vi "Modbus Master Simple.vi"() -> ()   [LabVIEW 2017]
uses:
  <vilib>/NI/Modbus Library/API/Master/Set Read Timeout.vi
  <vilib>/NI/Modbus Library/API/Read Transmission Data Unit.vi
  <vilib>/NI/Modbus Library/API/Write Transmission Data Unit.vi
  <vilib>/NI/Modbus Library/Transmission Data Unit/Write read operation timeout.vi
  <vilib>/NI/Modbus Library/API/Wrapper/Create Serial Master.vi
  <vilib>/NI/Modbus Library/API/Master/Modbus Master.lvclass
  <vilib>/NI/Modbus Library/API/Wrapper/API Main.lvlib
panel:
  in  "Read Timeout":i32=500
  out "Array 5":errorcluster[](array[cluster])
  in  "Inputs":T1(array[cluster])=[{"Inputs"=[0, 0, 0, 0], "Address"=0, "Number"=4}] {"Inputs" scale=0.0..65535.0}
  in  "Stop Button":bool
  out "Array 4":errorcluster[](array[cluster])
  out "Array 3":errorcluster[](array[cluster])
  out "Array 2":errorcluster[](array[cluster])
  out "Array":errorcluster[](array[cluster])=[{"status"=FALSE, "code"=0, "source"=""}, {"status"=TRUE, "code"=538183, "source"="<APPEND>Function 15"}, {"status"=TRUE, "code"=538183, "source"="<APPEND>Function 15"}]
  out "error out":errorcluster
  in  "Write Holding Reg":T2(array[cluster])=[{"Registers"=[1, 2], "Address"=4, "Number"=2}]
  in  "Read Holding Reg":T2(array[cluster])=[{"Registers"=[0, 0], "Address"=0, "Number"=2}]
  in  "DIscrete Inputs":T3(array[cluster])=[{"Inputs"=[TRUE, FALSE, TRUE, FALSE], "Address"=0, "Number"=4}]
  in  "Coils":cluster{"Coils":bool[], "Address":u16}[](array[cluster])=[{"Coils"=[TRUE, TRUE, TRUE, TRUE, TRUE], "Address"=0}, {"Coils"=[], "Address"=8}, {"Coils"=[], "Address"=16}] {"Address" format="%x"}
  in  "Update Period(ms)":u64=200
  in  "baud rate":u32=9600
  in  "VISA resource name":refnum<visa-resource-name>="COM13"
  in  "unit ID":u8=1
  in  "serial type":enum16{"RTU", "ASCII"}(ring)=enum."ASCII"
  in  "Connect":bool
  # "Slave"
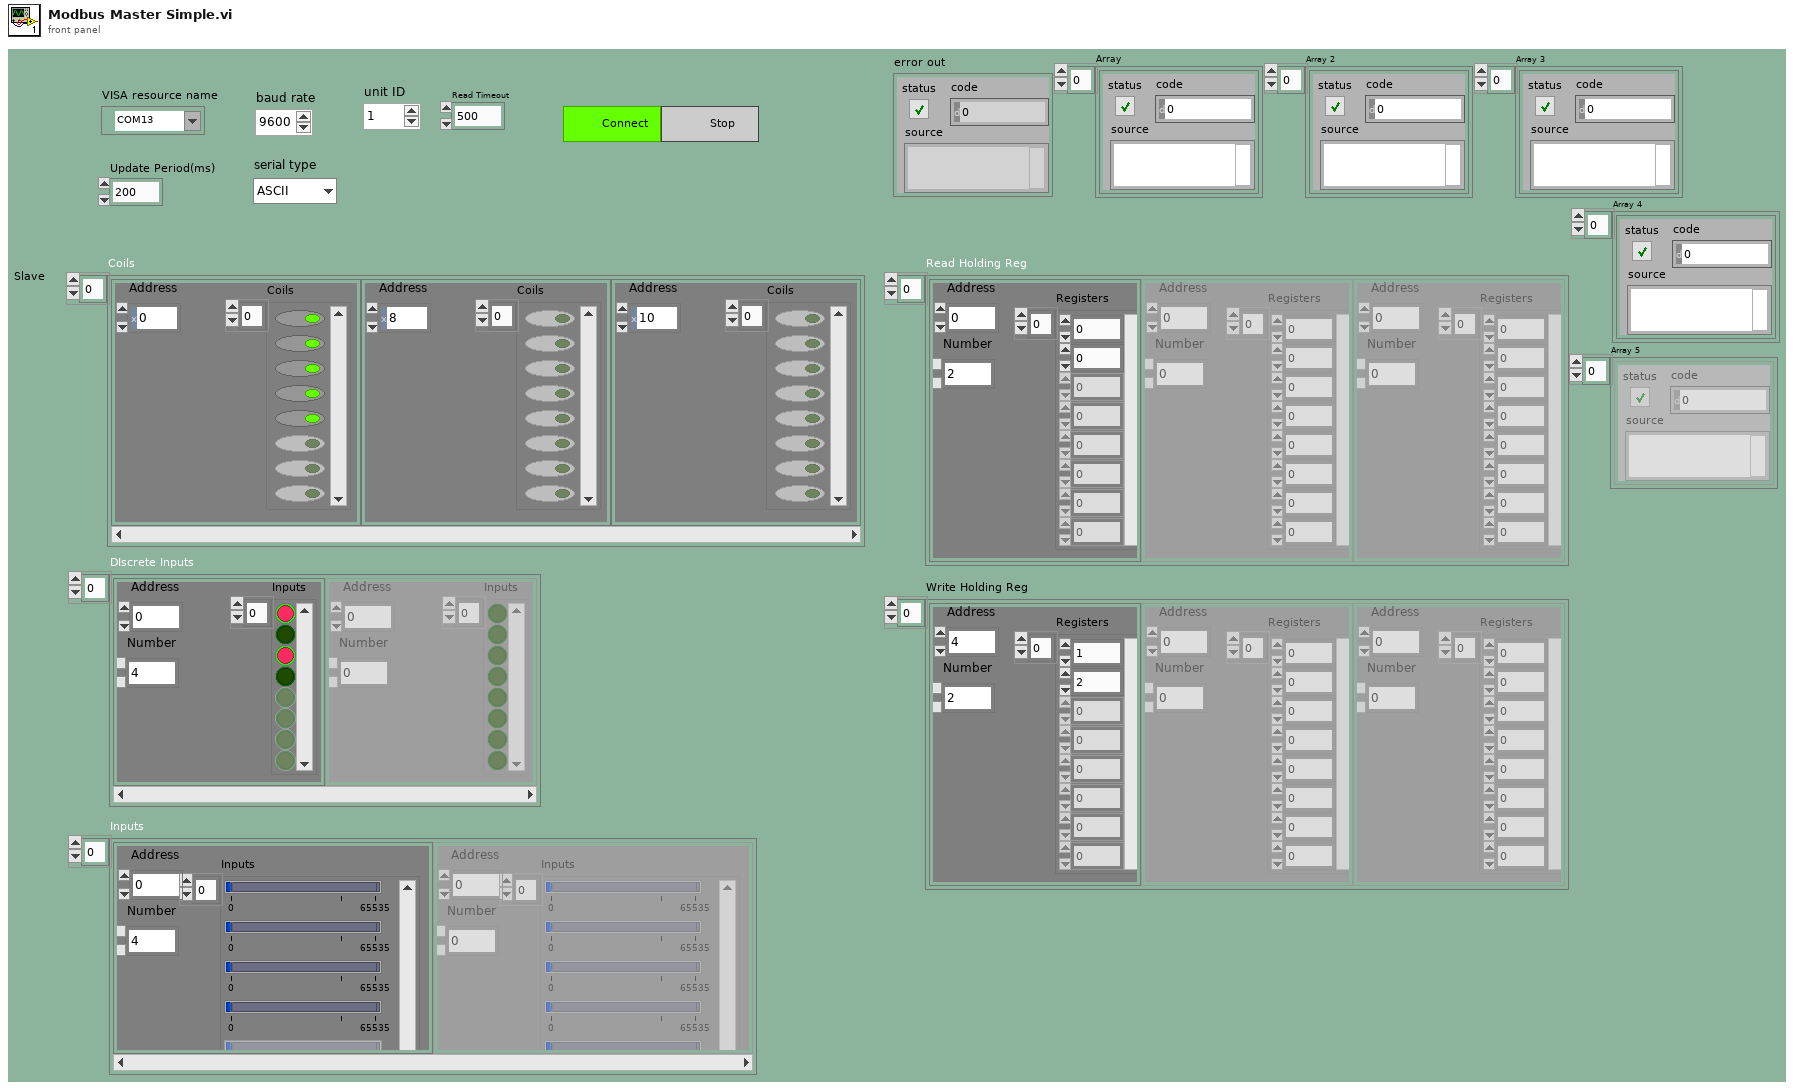
[diagram p1: front panel]
types:
  T1 = cluster{"Inputs":u16[], "Address":u16, "Number":u16}[]
  T2 = cluster{"Registers":u16[], "Address":u16, "Number":u16}[]
  T3 = cluster{"Inputs":bool[], "Address":u16, "Number":u16}[]
  T4 = cluster{"Inputs":bool[], "Address":u16, "Number":u16}
  T5 = cluster{"Inputs":u16[], "Address":u16, "Number":u16}
  T6 = cluster{"Registers":u16[], "Address":u16, "Number":u16}
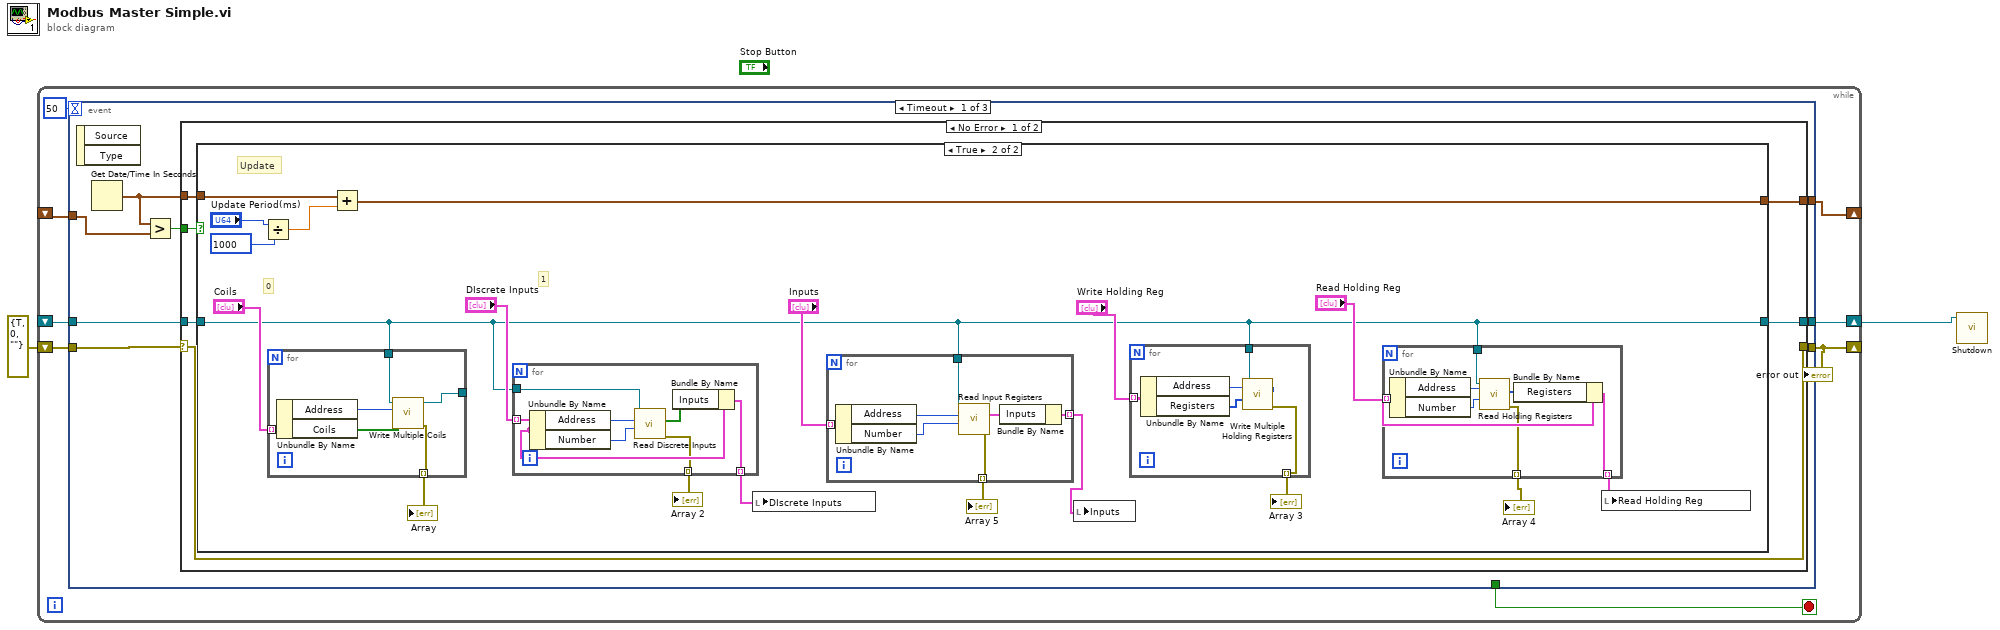
[diagram p0: block diagram]
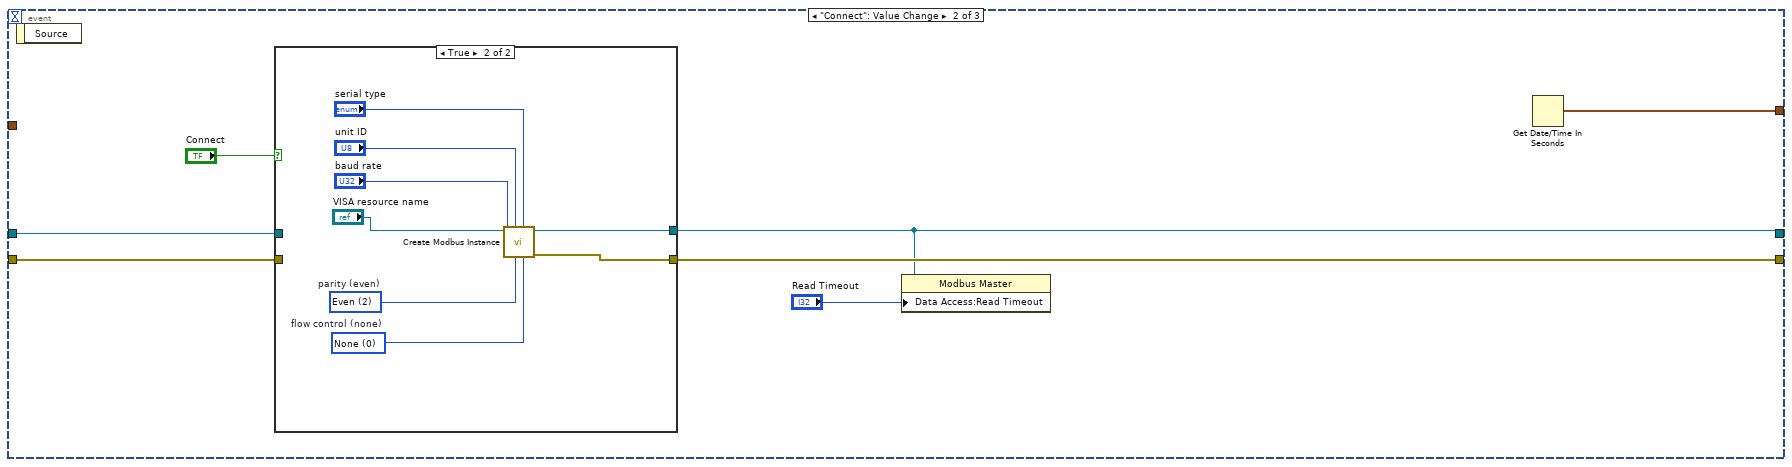
[diagram p4: hidden frame]
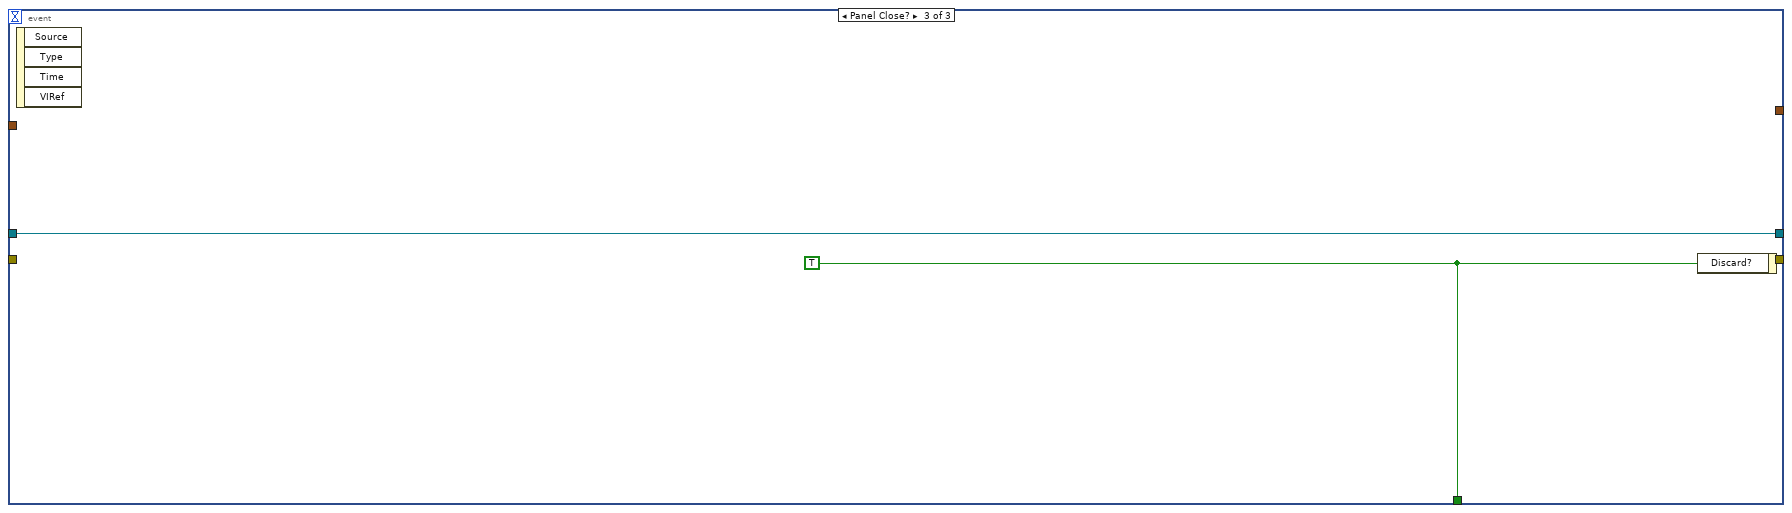
[diagram p6: hidden frame]
diagram:
  n1 = while {
    shift-right: [w10] -> w2
    shift-left: _ -> [w9]
    shift-right: [w6] -> _
    shift-left: _ -> [w7]
    shift-right: [w3] -> _
    shift-left: errorcluster {"status"=TRUE, "code"=0, "source"=""} ("error out") -> [w4]
    stop <- w5 stop-if-true
    n2 = event shown="[0] Timeout" {
      selector: _ -> [_ _ _]
      dyn-events: _ -> [_ _ _]
      timeout: 50 -> [_ _ _]
      tunnel: [w13 w82 w98] -> w10
      tunnel: w9 -> [w15 w86 w98]
      tunnel: w7 -> [w14 _ _]
      tunnel: [w16 w84 _] -> w6
      tunnel: [_ _ w99] -> w5
      tunnel: [w11 w85 _] -> w3
      tunnel: w4 -> [w12 w83 _]
      event Timeout {
        n3 = event-data() -> ()  [unwired: 1 in, 2 out]
        n4 = Get Date/Time In Seconds() -> (seconds since 1Jan1904=w17:timestamp)
        n5 = Greater?(x=w17, y=w14) -> (0:w18:bool)
        n6 = case shown="No Error" w12 {
          selector: w12 -> [w19 w78]
          tunnel: w18 -> [w24 _]
          tunnel: w17 -> [w23 w79]
          tunnel: [w22 w79] -> w16
          tunnel: w15 -> [w21 w80]
          tunnel: [w20 w80] -> w13
          tunnel: [w19 w78] -> w11
          frame No Error {
            n7 = case shown="True" w24 {
              tunnel: w23 -> [w26 w42]
              tunnel: [w26 w41] -> w22
              tunnel: w21 -> [w25 w29]
              tunnel: [w25 w29] -> w20
              frame False {
              }
              frame True {
                # "1"
                # "0"
                # "Update"
                n8 = Divide(x="Update Period(ms)", y=u64 1000) -> (x/y=w43:dbl)
                n9 = for {
                  tunnel: "Coils" -> [w77] mode=indexing
                  tunnel: [w74] -> _
                  tunnel: [w73] -> w34 mode=indexing
                  tunnel: w29 -> [w72]
                  n10 = Unbundle By Name(w77) -> ("Address"=w76:u16, "Coils"=w75:bool[])
                  n11 = call-dynamic "Write Multiple Coils.vi"("coils to write"=w75, "starting address"=w76, "Modbus master in"=w72) -> ("error out"=w73:errorcluster, "Modbus master out"=w74:refnum<class "Modbus Master.lvclass">)  [unwired: 7 in]
                }
                "Array" <- w34
                n12 = Add(x=w42, y=w43) -> (x+y=w41:timestamp)
                n13 = for {
                  tunnel: w29 -> [w71]
                  tunnel: "DIscrete Inputs" -> [w68] mode=indexing
                  tunnel: [w66] -> w38 mode=indexing
                  tunnel: [w65] -> w33 mode=indexing
                  n14 = Unbundle By Name(w68) -> ("Address"=w70:u16, "Number"=w69:u16)
                  n15 = call-dynamic "Read Discrete Inputs.vi"("number of inputs"=w69, "starting address"=w70, "Modbus master in"=w71) -> ("error out"=w65:errorcluster, "discrete inputs"=w67:bool[])  [unwired: 6 in, 1 out]
                  n16 = Bundle By Name(cluster=w68, "Inputs"=w67) -> (w66:T4)
                }
                "Array 2" <- w33
                n17 = local write "DIscrete Inputs"(w38) -> ()
                n18 = for {
                  tunnel: [w52] -> w27 mode=indexing
                  tunnel: "Inputs" -> [w48] mode=indexing
                  tunnel: w29 -> [w51]
                  tunnel: [w47] -> w28 mode=indexing
                  n19 = Unbundle By Name(w48) -> ("Address"=w50:u16, "Number"=w49:u16)
                  n20 = call-dynamic "Read Input Registers.vi"("number of inputs"=w49, "starting address"=w50, "Modbus master in"=w51) -> ("error out"=w52:errorcluster, "register values"=w46:u16[])  [unwired: 6 in, 1 out]
                  n21 = Bundle By Name(cluster=w48, "Inputs"=w46) -> (w47:T5)
                }
                "Array 5" <- w27
                n22 = local write "Inputs"(w28) -> ()
                n23 = for {
                  tunnel: "Write Holding Reg" -> [w64] mode=indexing
                  tunnel: w29 -> [w61]
                  tunnel: [w60] -> w32 mode=indexing
                  n24 = Unbundle By Name(w64) -> ("Address"=w63:u16, "Registers"=w62:u16[])
                  n25 = call-dynamic "Write Multiple Holding Registers.vi"("registers to write"=w62, "starting address"=w63, "Modbus master in"=w61) -> ("error out"=w60:errorcluster)  [unwired: 7 in, 1 out]
                }
                "Array 3" <- w32
                n26 = for {
                  tunnel: "Read Holding Reg" -> [w56] mode=indexing
                  tunnel: w29 -> [w58]
                  tunnel: [w54] -> w35 mode=indexing
                  tunnel: [w53] -> w31 mode=indexing
                  n27 = Unbundle By Name(w56) -> ("Address"=w59:u16, "Number"=w57:u16)
                  n28 = call-dynamic "Read Holding Registers.vi"("number of inputs"=w57, "starting address"=w59, "Modbus master in"=w58) -> ("error out"=w53:errorcluster, "register values"=w55:u16[])  [unwired: 6 in, 1 out]
                  n29 = Bundle By Name(cluster=w56, "Registers"=w55) -> (w54:T6)
                }
                "Array 4" <- w31
                n30 = local write "Read Holding Reg"(w35) -> ()
              }
            }
          }
          frame Error {
          }
        }
      }
      event "Connect": Value Change {
        n31 = event-data() -> ()  [unwired: 1 in, 1 out]
        n32 = case shown="True" "Connect" {
          tunnel: [w89 w91] -> w82
          tunnel: w86 -> [w89 _]
          tunnel: [w88 w90] -> w85
          tunnel: w83 -> [w88 _]
          frame False {
          }
          frame True {
            w96 = u16 0 items=["None", "XON/XOFF", "RTS/CTS", "XON/XOFF & RTS/CTS", "DTR/DSR", "XON/XOFF & DTR/DSR"]  # flow control (none)
            w94 = u16 2 items=["None", "Odd", "Even", "Mark", "Space"]  # parity (even)
            n33 = call-poly <vilib>:"Create Modbus Instance.vi"("flow control (none)"=w96, "serial type"="serial type", "parity (even)"=w94, "unit ID"="unit ID", "baud rate"="baud rate", "VISA resource name"="VISA resource name") -> ("error out"=w90:errorcluster, "serial master instance"=w91:refnum<class "Modbus Master.lvclass">)  [unwired: 4 in]
          }
        }
        n34 = property class="Modbus Master"(reference=w82, "Data Access:Read Timeout"="Read Timeout") -> ()  [unwired: 1 in, 2 out]
        n35 = Get Date/Time In Seconds() -> (seconds since 1Jan1904=w84:timestamp)
      }
      event Panel Close? {
        w99 = TRUE ("Discard?")
        n36 = event-data() -> ()  [unwired: 1 in, 4 out]
        n37 = event-data("Discard?"=w99) -> ()  [unwired: 1 in, 1 out]
      }
    }
    "error out" <- w3
  }
  n38 = call-dynamic "Shutdown.vi"("Modbus master in"=w2) -> ()  [unwired: 10 in, 1 out]
